vi "Append Text to Rich Text Box.vi"(8 "error in (no error)":errorcluster, 9 "Text Formatting":T1={"Font"="Default", "Text Color"=enum."Unchanged", "Text Background Color"=enum."Unchanged", "Text Style"=enum."Regular", "Font Size (Points)"=-1.0, "Text Alignment"=0} {"Text Alignment" items=["Left", "Right", "Center"]}, 10 "String":string="\r\nALiX stopped on 7/2/2016 at 12:14 PM\n\r\n", 11 ".NET Refnum in":refnum<k24>) -> (0 "Error Out":errorcluster, 2 "Rtf Content":string)   [LabVIEW 2019, in "Rich Text Box.lvlib"]
uses:
  Rich Text Box.lvlib
  System.Windows.Forms
  Text Formatting.ctl
  Text Colors.ctl
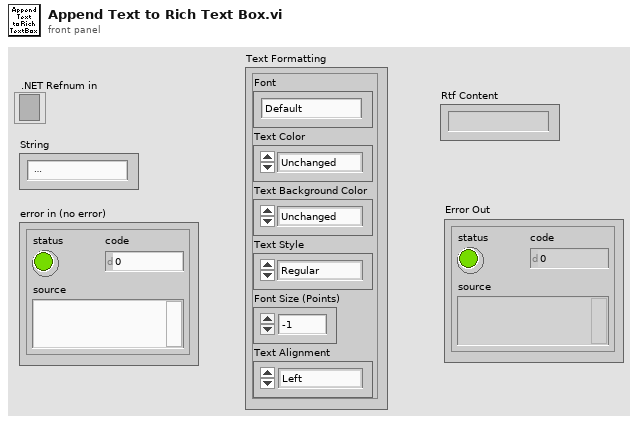
[diagram p1: front panel]
types:
  T1 = typedef "Rich Text Box.lvlib/Text Formatting.ctl" = cluster{"Font":string, "Text Color":T2, "Text Background Color":T2, "Text Style":enum16{"Regular", "Bold", "Italic", "Underline", "Strikeout"}, "Font Size (Points)":dbl, "Text Alignment":i32}
  T2 = typedef "Rich Text Box.lvlib/Text Colors.ctl" = enum16{"Unchanged", "Black", "Blue", "Brown", "Gray", "Green", "Orange", "Pink", "Red", "White"}
  T3 = enum16{"Regular", "Bold", "Italic", "Underline", "Strikeout"}
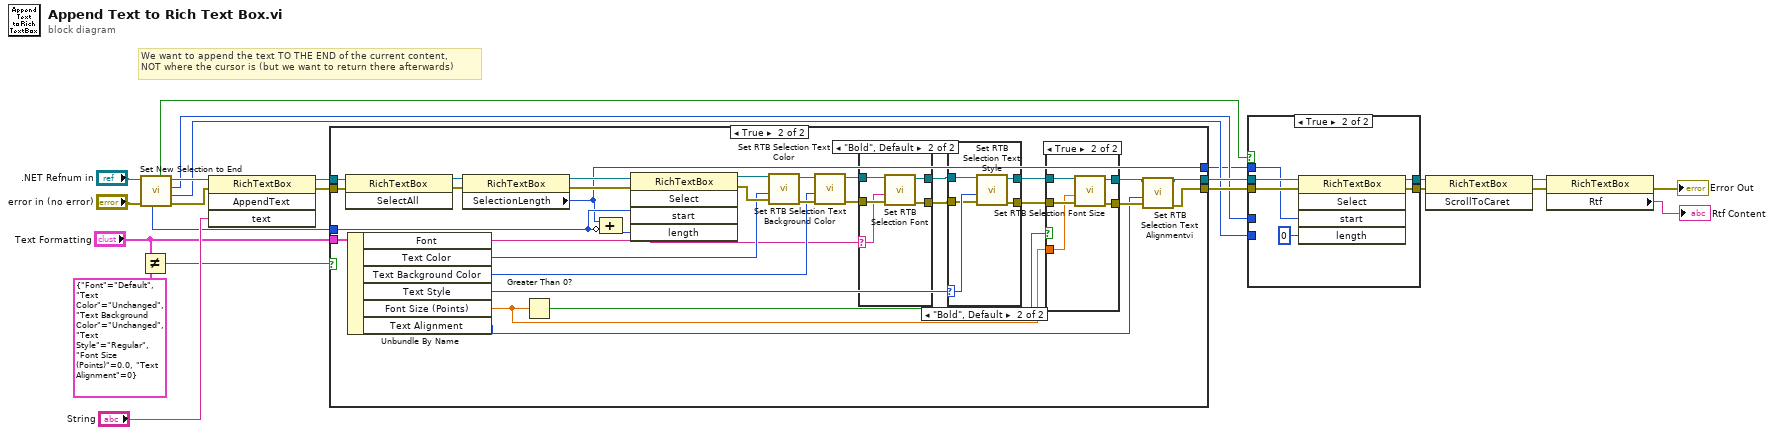
[diagram p0: block diagram]
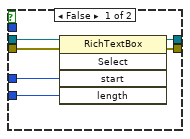
[diagram p2: hidden frame]
diagram:
  # "We want to append the text TO THE END of the current content,\nNOT where the cursor is (but we want to return there afterwards)"
  n1 = Not Equal?(x="Text Formatting", y=T1 {"Font"="Default", "Text Color"=enum."Unchanged", "Text Background Color"=enum."Unchanged", "Text Style"=enum."Regular", "Font Size (Points)"=0.0, "Text Alignment"=0} ("Text Formatting")) -> (x != y?=w10:bool)
  n2 = call "Set New Selection to End.vi"("error in (no error)"="error in (no error)", ".NET Refnum in"=".NET Refnum in") -> ("error out"=w19:errorcluster, "Current SelectionLength"=w8:i32, "Current SelectionStart"=w9:i32, ".NET Refnum out"=w20:refnum<k24>, "Current Selection at End?"=w6:bool, "New SelectionStart: End of RTB"=w7:i32)  [unwired: 4 in]
  n3 = invoke class="RichTextBox" method="AppendText"(reference=w20, error in=w19, "text"="String") -> (reference out=w18:refnum<k24>, error out=w17:errorcluster)  [unwired: 1 in, 2 out]
  n4 = case shown="True" w10 {
    tunnel: w18 -> [w26 w57]
    tunnel: w17 -> [w25 w56]
    tunnel: w7 -> [w24 w55]
    tunnel: "Text Formatting" -> [_ w54]
    tunnel: [w25 w30] -> w12
    tunnel: [w26 w29] -> w11
    tunnel: [w24 w27] -> w5
    frame False {
    }
    frame True {
      n5 = invoke class="RichTextBox" method="SelectAll"(reference=w57, error in=w56) -> (reference out=w53:refnum<k24>, error out=w52:errorcluster)  [unwired: 1 in, 1 out]
      n6 = Unbundle By Name(w54) -> ("Font"=w37:string, "Text Color"=w46:T2, "Text Background Color"=w43:T2, "Text Style"=w42:T3, "Font Size (Points)"=w38:dbl, "Text Alignment"=w28:i32)
      n7 = property class="RichTextBox"(reference=w53, error in=w52) -> (reference out=w51:refnum<k24>, error out=w50:errorcluster, "SelectionLength"=w27:i32)
      n8 = Greater Than 0?(x=w38) -> (x > 0?=w41:bool)
      n9 = Compound Arithmetic op=ADD(w27, invert w55) -> (w49:i32)
      n10 = invoke class="RichTextBox" method="Select"(reference=w51, error in=w50, "start"=w55, "length"=w49) -> (reference out=w48:refnum<k24>, error out=w47:errorcluster)  [unwired: 1 in, 3 out]
      n11 = call "Set RTB Selection Text Color.vi"("Error In"=w47, "Text Color"=w46, ".NET RTB Refnum in"=w48) -> ("Error Out"=w44:errorcluster, ".NET RTB Refnum out"=w45:refnum<k24>)  [unwired: 7 in]
      n12 = call "Set RTB Selection Text Background Color.vi"("Error In"=w44, "Text Background Color"=w43, ".NET RTB Refnum in"=w45) -> ("Error Out"=w35:errorcluster, ".NET RTB Refnum out"=w36:refnum<k24>)  [unwired: 7 in]
      n13 = case shown="\"Bold\", Default" w37 {
        selector: w37 -> [_ w60]
        tunnel: w36 -> [w59 w64]
        tunnel: w35 -> [w58 w63]
        tunnel: [w58 w62] -> w33
        tunnel: [w59 w61] -> w34
        frame "" {
        }
        frame "Bold", Default {
          n14 = call "Set RTB Selection Font.vi"("Error In"=w63, "Font Name"=w60, ".NET RTB Refnum in"=w64) -> ("Error Out"=w62:errorcluster, ".NET RTB Refnum out"=w61:refnum<k24>)  [unwired: 7 in]
        }
      }
      n15 = case shown="\"Bold\", Default" w42 {
        selector: w42 -> [_ w77]
        tunnel: w34 -> [w73 w78]
        tunnel: w33 -> [w72 w76]
        tunnel: [w72 w75] -> w39
        tunnel: [w73 w74] -> w40
        frame "Regular" {
        }
        frame "Bold", Default {
          n16 = call "Set RTB Selection Text Style.vi"("Error In"=w76, "Style"=w77, ".NET RTB Refnum in"=w78) -> ("Error Out"=w75:errorcluster, ".NET RTB Refnum out"=w74:refnum<k24>)  [unwired: 7 in]
        }
      }
      n17 = case shown="True" w41 {
        tunnel: w40 -> [w66 w71]
        tunnel: w39 -> [w65 w70]
        tunnel: [w65 w69] -> w31
        tunnel: [w66 w68] -> w32
        tunnel: w38 -> [_ w67]
        frame False {
        }
        frame True {
          n18 = call "Set RTB Selection Font Size.vi"("Error In"=w70, "Font Size (Points)"=w67, ".NET RTB Refnum in"=w71) -> ("Error Out"=w69:errorcluster, ".NET RTB Refnum out"=w68:refnum<k24>)  [unwired: 7 in]
        }
      }
      n19 = call "Set RTB Selection Text Alignmentvi.vi"("Error In"=w31, "Text Alignment"=w28, ".NET RTB Refnum in"=w32) -> ("Error Out"=w30:errorcluster, ".NET RTB Refnum out"=w29:refnum<k24>)  [unwired: 7 in]
    }
  }
  n20 = case shown="True" w6 {
    tunnel: [w84 w90] -> w22
    tunnel: [w83 w89] -> w21
    tunnel: w12 -> [w82 w88]
    tunnel: w11 -> [w81 w87]
    tunnel: w9 -> [w80 _]
    tunnel: w8 -> [w79 _]
    tunnel: w5 -> [_ w85]
    frame False {
      n21 = invoke class="RichTextBox" method="Select"(reference=w81, error in=w82, "start"=w80, "length"=w79) -> (reference out=w84:refnum<k24>, error out=w83:errorcluster)  [unwired: 1 in, 3 out]
    }
    frame True {
      n22 = invoke class="RichTextBox" method="Select"(reference=w87, error in=w88, "start"=w85, "length"=0) -> (reference out=w90:refnum<k24>, error out=w89:errorcluster)  [unwired: 1 in, 3 out]
    }
  }
  n23 = invoke class="RichTextBox" method="ScrollToCaret"(reference=w22, error in=w21) -> (reference out=w2:refnum<k24>, error out=w4:errorcluster)  [unwired: 1 in, 1 out]
  n24 = property class="RichTextBox"(reference=w2, error in=w4) -> (error out=→"Error Out":errorcluster, "Rtf"=→"Rtf Content":string)  [unwired: 1 out]
